vi "Gui_SetupProcessing.vi"(8 "error in (no error)":errorcluster, 11 "Variant":variant) -> (0 "error out":errorcluster caption="sortie d'erreur", 3 "Variant out":variant)   [LabVIEW 2018]
doc: "This VI setup the PROCESSING parameters.\n\n1. The PROCESSING parameters are passed by a Variant as input.\n2. Init the controls with the previous values.\n3. Wait for the user events, and update controls accordingly.\n4. When OK is pushed, return an updated Variant as output."
uses:
  controls/PROCESSING_Inputs.ctl
  controls/SEQUENCE_Inputs.ctl
  controls/EXCIT_Inputs.ctl
  controls/DATA_Inputs.ctl
  controls/TIMING_Inputs.ctl
  controls/TRAPPING_Inputs.ctl
panel:
  in  "SEQUENCE Inputs":T1={"EXCIT Inputs"={"Number of Excitations"=1, "Script Text"="", "Table of Waveforms"=[]}, "DATA Inputs"={"Record Length"=8192, "Sample Rate"=4.0, "Data Type"=0, "Vertical Range"=0.0, "Acquisition Duration"=100000.0}, "TIMING Inputs"={"Number of Acquisitions "=1, "Number of Accumulations"=1, "Table of Waveforms"=[], "Script Text"=""}, "PROCESSING Inputs"={"Reference Mass"=300.0939, "Cyclotron Freq"=255.727, "Magnetron Freq"=0.001}, "TRAPPING Inputs"={"Number of Channels"=4, "Init Values"=[2.0, 5.0, 5.0, 2.0], "Opening Values"=[0.0, 0.0, 0.0, 0.0], "Trapping Values"=[2.0, 5.0, 5.0, 2.0], "Emptying Values"=[-5.0, -5.0, -5.0, -5.0], "Adiabatic ON"=FALSE, "Adiabatic Duration"=0, "Adiabatic Waveforms"=["Adiabatic_None_2_2_2000.bin", "Adiabatic_Ramp_5_0_2000.bin", "Adiabatic_DoubleRamp_5_0_2000.bin", "Adiabatic_RC_2_0_2000.bin"], "Ions Refill ON"=FALSE, "Number of Ions Refills"=4, "Trapping Delay"=400.0, "Trapping Duration"=300.0}} {"TRAPPING Inputs"."Trapping Duration" min=2.0; "TRAPPING Inputs"."Trapping Delay" min=2.0; "TRAPPING Inputs"."Number of Ions Refills" min=1 max=1000; "TRAPPING Inputs"."Trapping Values" min=-10.0 max=10.0; "TRAPPING Inputs"."Init Values" min=-10.0 max=10.0; "TRAPPING Inputs"."Emptying Values" min=-10.0 max=10.0; "TRAPPING Inputs"."Opening Values" min=-10.0 max=10.0; "PROCESSING Inputs"."Magnetron Freq" format="%.5g"; "PROCESSING Inputs"."Cyclotron Freq" format="%.5g"; "PROCESSING Inputs"."Reference Mass" format="%.5g"; "TIMING Inputs"."Number of Accumulations" min=0 max=50 step=1; "TIMING Inputs"."Number of Acquisitions" min=1 max=10 step=1; "DATA Inputs"."Vertical Range" items=["0.2"=0.2, "0.4"=0.4, "1"=1.0, "2"=2.0, "4"=4.0, "10"=10.0]; "DATA Inputs"."Data Type" items=["I16", "DBL"]; "DATA Inputs"."Sample Rate" items=["1 MHz"=1000000.0, "2 MHz"=2000000.0, "5 MHz"=5000000.0, "10 MHz"=10000000.0, "20 MHz"=20000000.0, "25 MHz"=25000000.0, "50 MHz"=50000000.0, "100 MHz"=100000000.0]; "EXCIT Inputs"."Number of Excitations" min=1 max=10}
  in  "PROCESSING Inputs":T5={"Reference Mass"=300.0939, "Cyclotron Freq"=255.727, "Magnetron Freq"=0.001} caption="DATA Inputs" {"Magnetron Freq" format="%.5g"; "Cyclotron Freq" format="%.5g"; "Reference Mass" format="%.5g"}
  in  "OK":bool
  # "GO_out"
  # "Gout"
  # "GI_in"
  # "Gin"
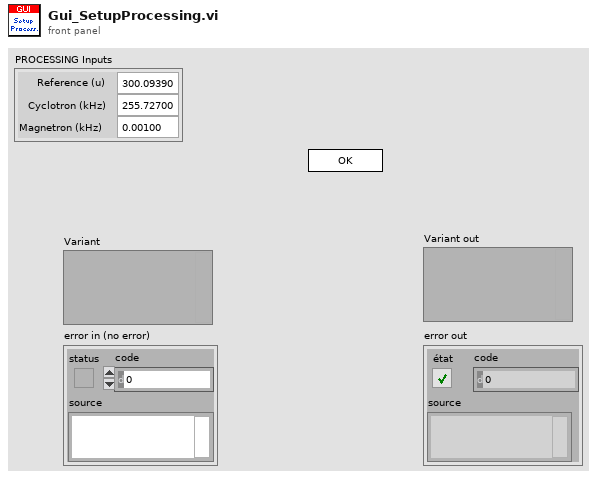
[diagram p1: front panel]
types:
  T1 = typedef "SEQUENCE_Inputs.ctl" = cluster{"EXCIT Inputs":T2, "DATA Inputs":T3, "TIMING Inputs":T4, "PROCESSING Inputs":T5, "TRAPPING Inputs":T6}
  T2 = typedef "EXCIT_Inputs.ctl" = cluster{"Number of Excitations":i32, "Script Text":string, "Table of Waveforms":string[]}
  T3 = typedef "DATA_Inputs.ctl" = cluster{"Record Length":i32, "Sample Rate":dbl, "Data Type":u8, "Vertical Range":dbl, "Acquisition Duration":dbl}
  T4 = typedef "TIMING_Inputs.ctl" = cluster{"Number of Acquisitions ":i16, "Number of Accumulations":i16, "Table of Waveforms":string[], "Script Text":string}
  T5 = typedef "PROCESSING_Inputs.ctl" = cluster{"Reference Mass":dbl, "Cyclotron Freq":dbl, "Magnetron Freq":dbl}
  T6 = typedef "TRAPPING_Inputs.ctl" = cluster{"Number of Channels":i32, "Init Values":dbl[], "Opening Values":dbl[], "Trapping Values":dbl[], "Emptying Values":dbl[], "Adiabatic ON":bool, "Adiabatic Duration":i32, "Adiabatic Waveforms":string[], "Ions Refill ON":bool, "Number of Ions Refills":i32, "Trapping Delay":dbl, "Trapping Duration":dbl}
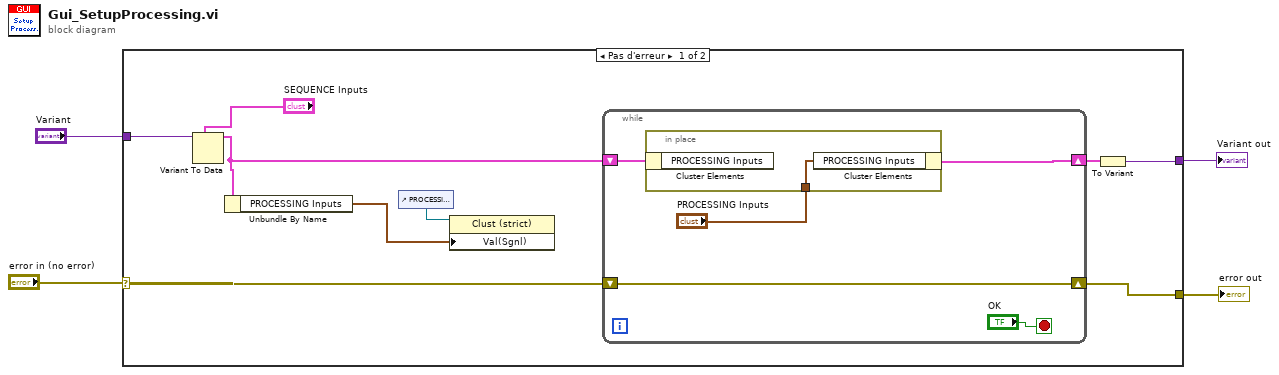
[diagram p0: block diagram]
diagram:
  n1 = case shown="Pas d'erreur" "error in (no error)" {
    selector: "error in (no error)" -> [w13 w21]
    tunnel: [w12 w21] -> w3
    tunnel: "Variant" -> [w10 w20]
    tunnel: [w7 w20] -> w1
    frame No Error {
      n2 = Variant To Data(type="SEQUENCE Inputs", Variant=w10) -> (data=w9:T1)  [unwired: 1 in, 1 out]
      n3 = Unbundle By Name(w9) -> ("PROCESSING Inputs"=w6:T5)
      n4 = control-ref of="PROCESSING Inputs"() -> (w5:refnum<vi>)
      n5 = property class="Clust (strict)"(reference=w5, "Val(Sgnl)"=w6) -> ()  [unwired: 1 in, 2 out]
      n6 = while {
        shift-right: [w18] -> w12
        shift-left: w13 -> [w18]
        shift-right: [w16] -> w8
        shift-left: w9 -> [w17]
        stop <- "OK" stop-if-true
        n7 = in-place {
          in-place-border: "PROCESSING Inputs" -> [w19]
          n8 = in-place-cluster #1(w17) -> ()  [unwired: 1 out]
          n9 = in-place-cluster #1("PROCESSING Inputs"=w19) -> (w16:T1)
        }
      }
      n10 = To Variant(anything=w8) -> (Variant=w7:variant)
    }
    frame Error {
    }
  }
  "error out" <- w3
  "Variant out" <- w1
